vi "Filter Banks - 2D.vi"() -> ()   [LabVIEW 2023]
doc: "This example shows how to acquire the detail coefficients and the approximation coefficients of an image with the WA Analysis Filter Bank VI. This example also shows how to reconstruct the image from the detail coefficients and the approximation coefficients with the WA Synthesis Filter Bank VI.\n\n<b>Instructions:</b>\n1) Run this VI.\n2) Observe the sub-band outputs of the image.\n3) Browse the Block Diagram to learn how to use the WA Analysis Filter Bank VI to perform one-level decomposition on an image, how to use the WA Synthesis Filter Bank VI to reconstruct the image, and how to use the WA Wavelet Filter VI to read analysis filters and synthesis filters of a wavelet."
uses:
  <vilib>/addons/Wavelet Analysis/filter banks.llb/WA 2D Analysis Filter Bank.vi
  <vilib>/addons/Wavelet Analysis/filter banks.llb/WA 2D Synthesis Filter Bank.vi
  <vilib>/addons/_Advanced Signal Processing/NI_AdvSigProcWA.lvlib
panel:
  in  "Data":u16(ring)=134 items=["1D Example Data"=100, "-"=101, "Doppler"=102, "HOP"=103, "TF Sine"=104, "Noisy Doppler"=105, "Sea Temperature"=106, "Sp500"=107, "Power Line"=108, "Engine Knocking"=109, "HeaviSine"=110, "Bumps"=111, "Blocks"=112, "Piece Regular"=113, "HypChirps"=114, "LinChirps"=115, "Chirps"=116, "Piece Polynomial"=117, "ECG"=131, "-"=118, "2D Example Data"=119, "-"=120, "Finger Print (Image)"=121, "Iris Flower (Image)"=122, "Mammogram (Image)"=123, "Lake (Image)"=127, "Two Can 1 (Image)"=132, "Two Can 2 (Image)"=133, "Camera Man (Image)"=134]
  out "Size 2(s)":i32[](array[numeric])
  out "Size 6(s)":i32[](array[numeric])
  out "Size 5(s)":i32[](array[numeric])
  out "Size 4(s)":i32[](array[numeric])
  out "Size 1(s)":i32[](array[numeric])
  out "Size 3(s)":i32[](array[numeric])
  out "High_High":dbl[][](graph)
  out "High_Low":dbl[][](graph)
  out "Low_High":dbl[][](graph)
  out "Low_Low":dbl[][](graph)
  out "Reconstructed Image":dbl[][](graph)
  out "Original Image":u8[][](graph)
  in  "Wavelet":u16(ring) items=["db02"=0, "db03"=1, "db04"=2, "db05"=3, "db06"=4, "db07"=5, "db08"=6, "db09"=7, "db10"=8, "db11"=9, "db12"=10, "db13"=11, "db14"=12, "Haar"=13, "bior1_3"=14, "bior1_5"=15, "bior2_2"=16, "bior2_4"=17, "bior2_6"=18, "bior2_8"=19, "bior3_1"=20, "bior3_3"=21, "bior3_5"=22, "bior3_7"=23, "bior3_9"=24, "bior4_4 (FBI)"=25, "bior5_5"=38, "bior6_8"=39, "coif1"=26, "coif2"=27, "coif3"=28, "coif4"=29, "coif5"=30, "sym2"=31, "sym3"=32, "sym4"=33, "sym5"=34, "sym6"=35, "sym7"=36, "sym8"=37]
  in  "Extension":u16(ring)=2 items=["Zero padding", "Symmetric", "Periodic", "Spline"]
  # "Overview: Shows how to acquire the detail coefficients and the approximation coefficients of an image with the WA Analysis Filter Bank VI.\nRequirements: LabVIEW Full Development System, Advanced Signal Processing Toolkit\nInstructions: \n1. Run this VI.\n2. Observe the sub-band outputs of the image.\n3. Browse the block diagram to learn how to use the WA Analysis Filter Bank VI to perform one-level decomposition on an image, how to use the WA Synthesis Filter Bank VI to reconstruct the image, and how to use the WA Wavelet Filter VI to read analysis filters and synthesis filters of a wavelet."
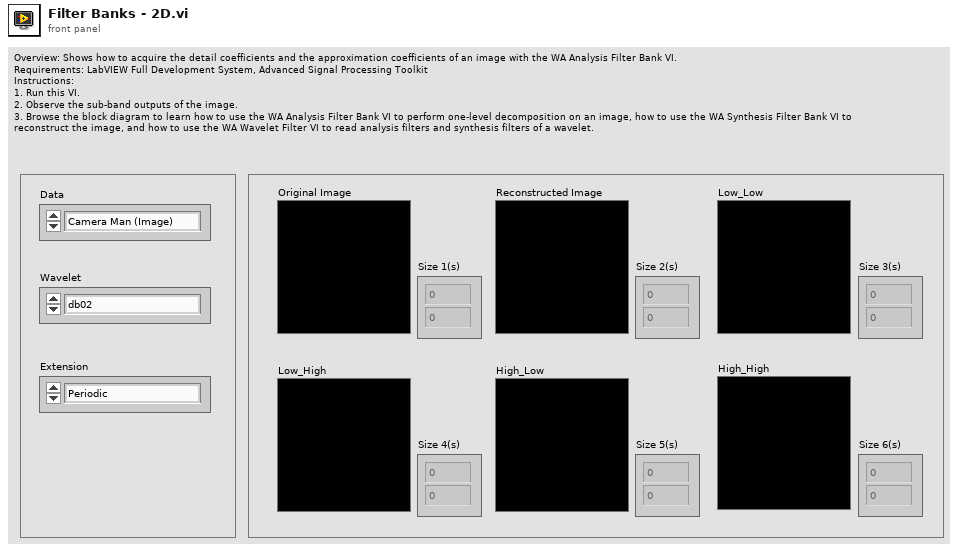
[diagram p1: front panel]
types:
  T1 = cluster{"low_low":dbl[][], "low_high":dbl[][], "high_low":dbl[][], "high_high":dbl[][]}
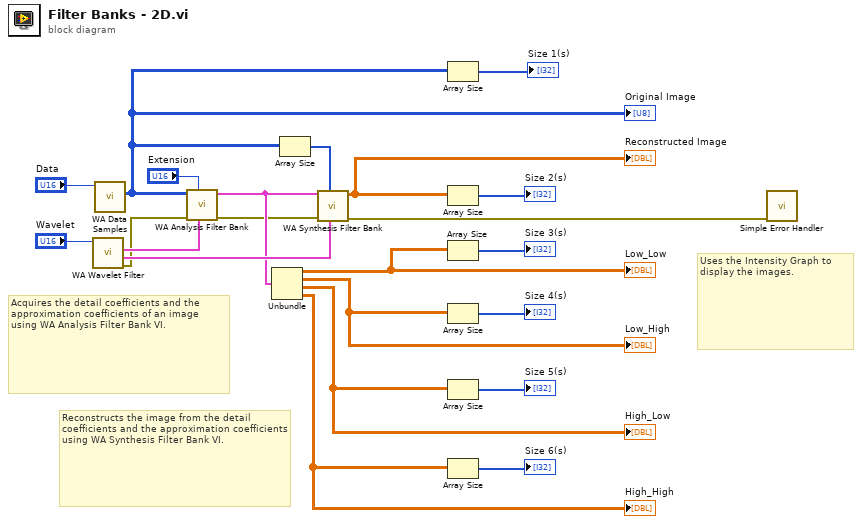
[diagram p0: block diagram]
diagram:
  # "Uses the Intensity Graph to display the images."
  # "Reconstructs the image from the detail coefficients and the approximation coefficients using WA Synthesis Filter Bank VI."
  # "Acquires the detail coefficients and the approximation coefficients of an image using WA Analysis Filter Bank VI."
  n1 = call <vilib>:"WA Wavelet Filter.vi"("wavelet"="Wavelet") -> ("error out"=w2:errorcluster, "synthesis filters"=w20:cluster{"lowpass":dbl[], "highpass":dbl[]}, "analysis filters"=w21:cluster{"lowpass":dbl[], "highpass":dbl[]})  [unwired: 3 in, 5 out]
  n2 = call <vilib>:"WA Data Samples.vi"("data"="Data") -> ("image"=w15:u8[][])  [unwired: 10 out]
  "Original Image" <- w15
  n3 = call-poly <vilib>:"WA Analysis Filter Bank.vi"("analysis filters"=w21, "extension"="Extension", "error in (no error)"=w2, "signal"=w15) -> ("error out"=w16:errorcluster, "DWT coef"=w17:T1)  [unwired: 6 out]
  n4 = Unbundle(w17) -> ("low_low"=w14:dbl[][], "low_high"=w1:dbl[][], "high_low"=w8:dbl[][], "high_high"=w7:dbl[][])
  "Low_Low" <- w14
  "Low_High" <- w1
  "High_Low" <- w8
  "High_High" <- w7
  n5 = Array Size(array=w15) -> (size(s)=w19:i32[])
  n6 = call-poly <vilib>:"WA Synthesis Filter Bank.vi"("synthesis filters"=w20, "size"=w19, "error in (no error)"=w16, "DWT coef"=w17) -> ("error out"=w3:errorcluster, "signal"=w5:dbl[][])  [unwired: 6 out]
  "Reconstructed Image" <- w5
  n7 = Array Size(array=w15) -> (size(s)=→"Size 1(s)":i32[])
  n8 = Array Size(array=w5) -> (size(s)=→"Size 2(s)":i32[])
  n9 = Array Size(array=w14) -> (size(s)=→"Size 3(s)":i32[])
  n10 = Array Size(array=w1) -> (size(s)=→"Size 4(s)":i32[])
  n11 = Array Size(array=w8) -> (size(s)=→"Size 5(s)":i32[])
  n12 = Array Size(array=w7) -> (size(s)=→"Size 6(s)":i32[])
  n13 = call <vilib>:"Simple Error Handler.vi"("error in (no error)"=w3) -> ()  [unwired: 4 in, 5 out]
